vi "niRFUtil FWK Configure Acquisition Timing.vi"(3 "Measurement Delay (0 sec)":dbl format="%^.2e", 4 "Desired Delay (0 sec)":dbl format="%^.2e", 5 "Desired Time (sec)":dbl=0.001 format="%^.2e") -> (0 "Measurement Delay (sec)":dbl format="%^.2e", 1 "Delay (sec)":dbl format="%^.2e", 2 "Time (sec)":dbl format="%^.2e")   [LabVIEW 2015, in "niRFUtil.lvlib"]
doc: "(c) Copyright 2006, National Instruments, Inc. This VI may not be duplicated, sold, or distributed without written consent from National Instruments."
uses:
  niRFUtil.lvlib
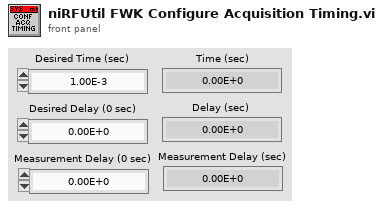
[diagram p1: front panel]
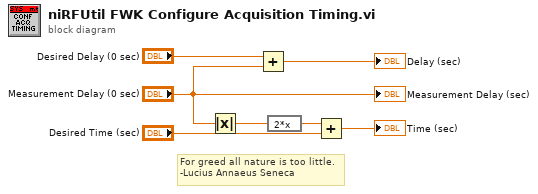
[diagram p0: block diagram]
diagram:
  # "For greed all nature is too little.\n-Lucius Annaeus Seneca"
  n1 = Absolute Value(x="Measurement Delay (0 sec)") -> (abs(x)=w5:dbl)
  n2 = Add(x="Desired Delay (0 sec)", y="Measurement Delay (0 sec)") -> (x+y=→"Delay (sec)":dbl)
  n3 = expression code="2*x"(w5) -> (w3:dbl)
  n4 = Add(x=w3, y="Desired Time (sec)") -> (x+y=→"Time (sec)":dbl)
  "Measurement Delay (sec)" <- "Measurement Delay (0 sec)"
